vi "Do.vi"(8 "error in (no error)":errorcluster, 11 "Open Form Button in":refnum<class "Open Form Button.lvclass">) -> (0 "error out":errorcluster, 3 "Open Form Button out":refnum<class "Open Form Button.lvclass">)   [LabVIEW 2020, in "Panel Form Controller.lvlib" / "Open Form Button.lvclass"]
uses:
  Open Form Button.lvclass
  Open Form Button.lvclass/Open Form Button.ctl
  Forms Model/Form Model Interfaces/Form Model Messages Messages/Open Form Msg/Open Form Msg.lvclass/Open Form Msg.ctl
  <vilib>/ActorFramework/Message Enqueuer/Message Enqueuer.lvclass/Message Enqueuer.ctl
  <vilib>/ActorFramework/Message Enqueuer/Enqueue.vi
  Forms Model/Form Model Interfaces/Form Model Messages Messages/Open Form Msg/Open Form Msg.lvclass
  C:/Program Files (x86)/National Instruments/LabVIEW 2020/vi.lib/ActorFramework/Message/Message.lvclass
  <vilib>/ActorFramework/Message Priority Queue/Priority Enqueue.vi
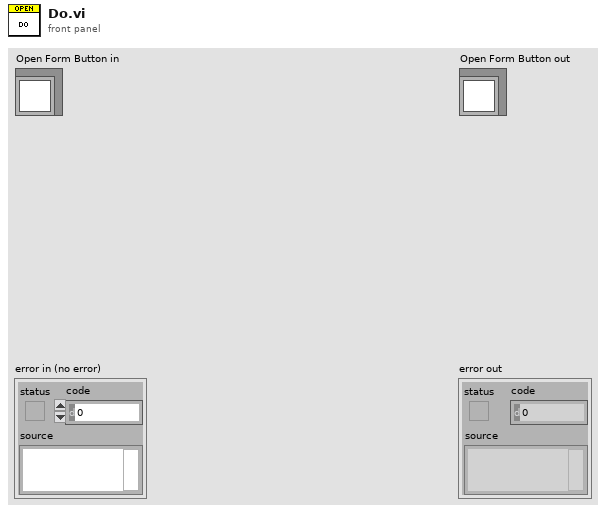
[diagram p1: front panel]
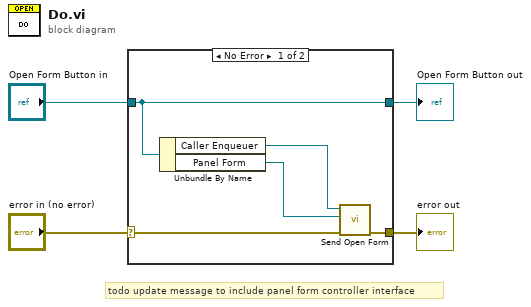
[diagram p0: block diagram]
diagram:
  # "todo update message to include panel form controller interface"
  n1 = case shown="No Error" "error in (no error)" {
    selector: "error in (no error)" -> [w9 w10]
    tunnel: [w8 w10] -> w3
    tunnel: "Open Form Button in" -> [w7 w11]
    tunnel: [w7 w11] -> w1
    frame No Error {
      n2 = Unbundle By Name(w7) -> ("Caller Enqueuer"=w6:refnum<class "Message Enqueuer.lvclass">, "Panel Form"=w5:refnum<class "Panel Form Controller.lvclass">)
      n3 = call "Send Open Form.vi"("error in (no error)"=w9, "Panel Form Controller"=w5, "Message Enqueuer"=w6) -> ("error out"=w8:errorcluster)  [unwired: 7 in, 1 out]
    }
    frame Error {
    }
  }
  "error out" <- w3
  "Open Form Button out" <- w1
